vi "getStringBounds.vi"(0 "reference":refnum<class "SegmentedLineEdge.lvclass">, 1 "graphics":refnum<class "Graphics.lvclass">, 2 "p1":T2 {"y" format="%.2f"; "x" format="%.2f"}, 3 "p2":T2 {"y" format="%.2f"; "x" format="%.2f"}, 4 "text":string, 5 "error in (no error)":errorcluster, 7 "center":bool) -> (14 "reference out":refnum<class "SegmentedLineEdge.lvclass">, 15 "bounds":T1 {"height" format="%.2f"; "width" format="%.2f"; "y" format="%.2f"; "x" format="%.2f"}, 19 "error out":errorcluster)   [LabVIEW 2016, in "SegmentedLineEdge.lvclass"]
doc: "\"public static Rectangle2D getStringBounds(Graphics2D g2,"
uses:
  <resource>/Framework/Providers/Open_GDS/UML/SegmentedLineEdge_class/SegmentedLineEdge.lvclass
  <resource>/Framework/Providers/Open_GDS/UML/General/Point/Point Point2D.ctl
  <resource>/Framework/Providers/Open_GDS/UML/Graphics_class/Graphics.lvclass
  <resource>/Framework/Providers/Open_GDS/UML/General/Rectangle/Rectangle Rectangle2D.ctl
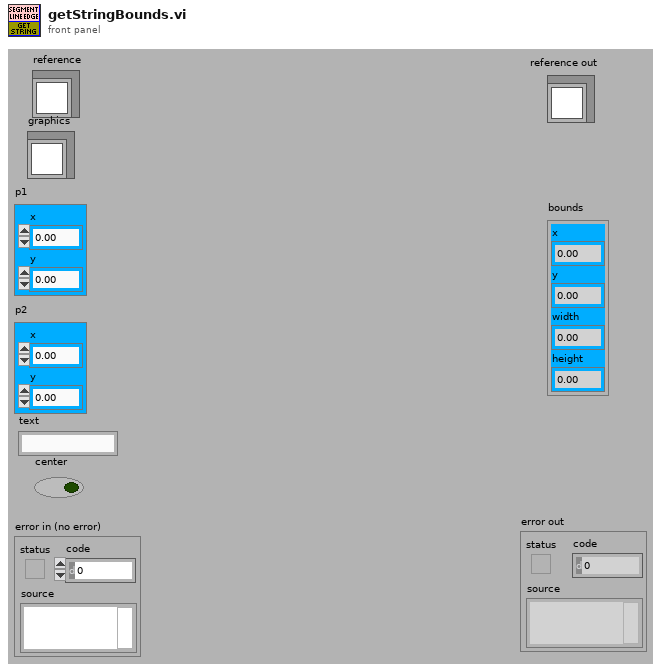
[diagram p1: front panel]
types:
  T1 = typedef "Rectangle Rectangle2D.ctl" = cluster{"x":dbl, "y":dbl, "width":dbl, "height":dbl}
  T2 = typedef "Point Point2D.ctl" = cluster{"x":dbl, "y":dbl}
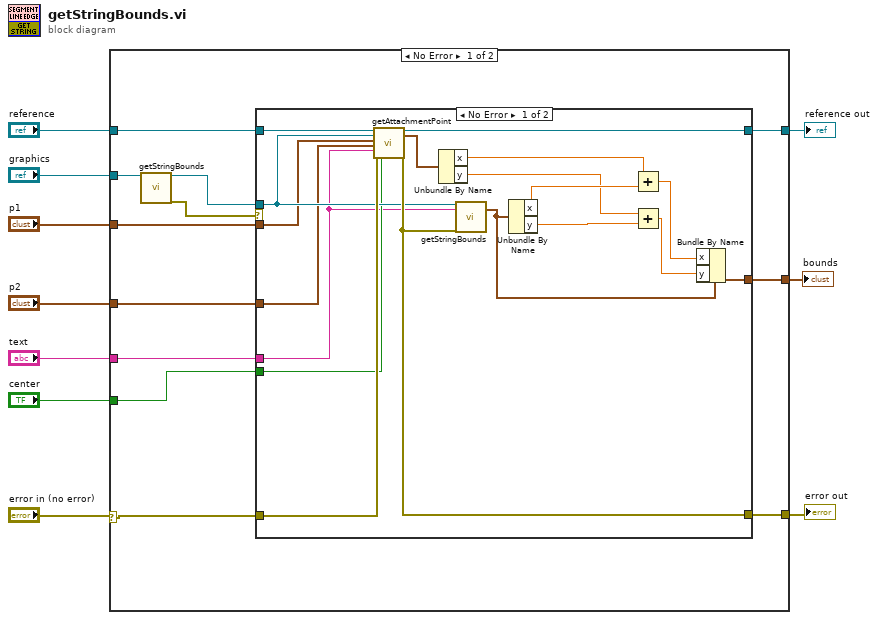
[diagram p0: block diagram]
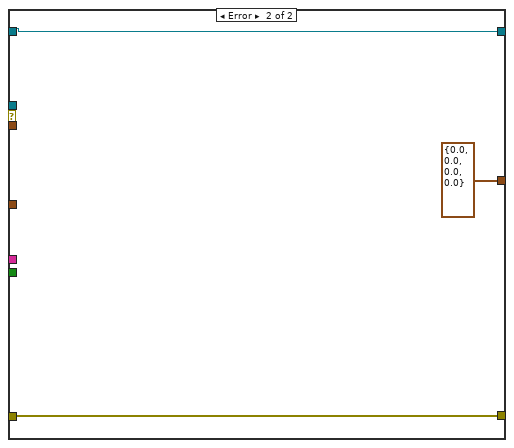
[diagram p2: hidden frame]
diagram:
  n1 = case shown="No Error" "error in (no error)" {
    selector: "error in (no error)" -> [w14 w44]
    tunnel: "reference" -> [w22 w45]
    tunnel: [w21 w44] -> w9
    tunnel: [w20 w45] -> w8
    tunnel: "graphics" -> [w13 _]
    tunnel: "p1" -> [w19 _]
    tunnel: "p2" -> [w18 _]
    tunnel: "text" -> [w17 _]
    tunnel: "center" -> [w16 _]
    tunnel: [w15 _] -> w1
    frame No Error {
      n2 = call-dynamic "getStringBounds.vi"("reference"=w13) -> ("reference out"=w12:refnum<class "Graphics.lvclass">, "error out"=w11:errorcluster)  [unwired: 16 in, 1 out]
      n3 = case shown="No Error" w11 {
        tunnel: [w40 w42] -> w20
        tunnel: [w37 w41] -> w21
        tunnel: w14 -> [w39 w41]
        tunnel: w22 -> [w38 w42]
        tunnel: [w26 T1 {"x"=0.0, "y"=0.0, "width"=0.0, "height"=0.0} ("bounds")] -> w15
        tunnel: w12 -> [w36 _]
        tunnel: w19 -> [w35 _]
        tunnel: w18 -> [w34 _]
        tunnel: w17 -> [w32 _]
        tunnel: w16 -> [w33 _]
        frame No Error {
          n4 = call-dynamic "getAttachmentPoint.vi"("reference"=w38, "graphics"=w36, "p1"=w35, "p2"=w34, "text"=w32, "error in (no error)"=w39, "center"=w33) -> ("reference out"=w40:refnum<class "SegmentedLineEdge.lvclass">, "attachPoint"=w28:T2, "error out"=w37:errorcluster)  [unwired: 10 in]
          n5 = Unbundle By Name(w28) -> ("x"=w31:dbl, "y"=w25:dbl)
          n6 = call-dynamic "getStringBounds.vi"("reference"=w36, "text"=w32, "error in (no error)"=w37) -> ("bounds"=w27:T1)  [unwired: 14 in, 2 out]
          n7 = Unbundle By Name(w27) -> ("x"=w30:dbl, "y"=w24:dbl)
          n8 = Add(x=w31, y=w30) -> (x+y=w29:dbl)
          n9 = Add(x=w25, y=w24) -> (x+y=w23:dbl)
          n10 = Bundle By Name(cluster=w27, "x"=w29, "y"=w23) -> (w26:T1)
        }
        frame Error {
        }
      }
    }
    frame Error {
    }
  }
  "reference out" <- w8
  "error out" <- w9
  "bounds" <- w1
